vi "Sub04_PosTxt.vi"(8 "error in (no error)":errorcluster, 11 "Application Directory":path) -> (0 "error out":errorcluster, 3 "String":string)   [LabVIEW 2019]
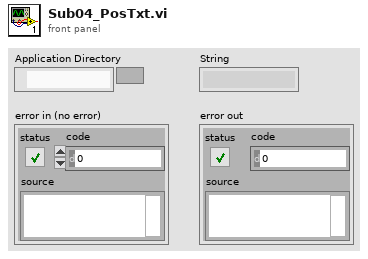
[diagram p1: front panel]
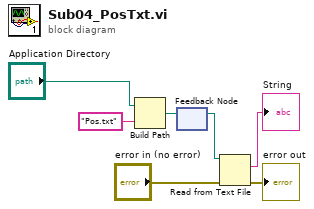
[diagram p0: block diagram]
diagram:
  n1 = Build Path(base path="Application Directory", name or relative path="Pos.txt") -> (appended path=w3:path)
  n2 = feedback #1() -> (w4:path)  [unwired: 1 in]
  n3 = feedback-in #1(w3) -> ()
  n4 = Read from Text File(file (use dialog)=w4, error in="error in (no error)") -> (text=→"String":string, error out=→"error out":errorcluster)  [unwired: 2 in, 2 out]
